vi "CoreState_Init.vi"(8 "error in (no error)":errorcluster, 11 "launcher in":refnum<class "launcher.lvclass">) -> (0 "error out":errorcluster, 3 "launcher out":refnum<class "launcher.lvclass">)   [LabVIEW 2021, in "launcher.lvclass"]
uses:
  launcher.lvclass
  TypeDefs/dvr_type.ctl
  _PARMS.ctl
  <userlib>/S2 Labs/Module Framework/Modules/Base/Launch Module Typdef.ctl
  <userlib>/S2 Labs/Module Framework/Modules/Base/Launch Module Parms.ctl
  launcher.lvclass/launcher.ctl
  <userlib>/S2 Labs/Module Framework/Modules/Base/Module.lvclass
  <userlib>/S2 Labs/Alarms and Events Toolkit/Alarms/Alarms Events.lvclass
  <vilib>/nisyscfg/nisyscfg.lvlib
  <resource>/objmgr/nisysapi.rc
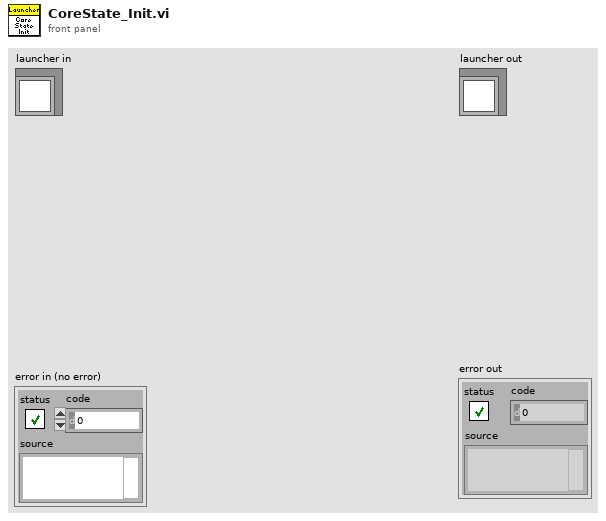
[diagram p1: front panel]
types:
  T1 = typedef "launcher.lvclass/dvr_type.ctl" = cluster{"_PARMS":T2}
  T2 = typedef "launcher.lvclass/_PARMS.ctl" = cluster{"ch_alias":string[], "ch_units":string[], "Modules to Launch":T3[]}
  T3 = typedef "Module.lvclass/Launch Module Typdef.ctl" = cluster{"Module":string, "Parameters":T4}
  T4 = typedef "Module.lvclass/Launch Module Parms.ctl" = cluster{"Name":string, "Arguments":string[], "Show FP?":bool}
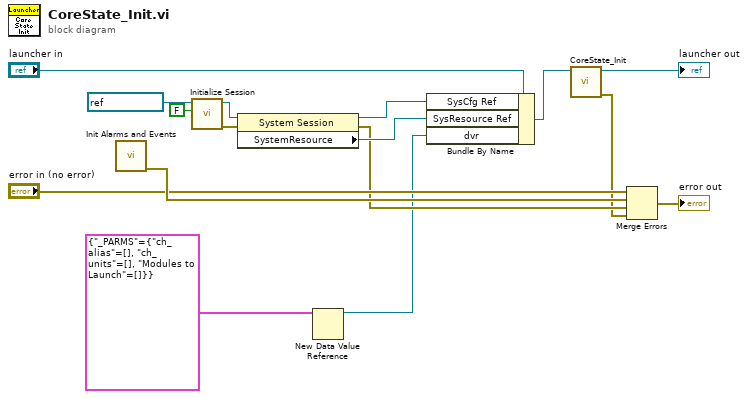
[diagram p0: block diagram]
diagram:
  n1 = call <userlib>:"Init Alarms and Events.vi"() -> ("error out"=w14:errorcluster)  [unwired: 11 in]
  n2 = call <vilib>:"Initialize Session.vi"("Force Property Refresh (T)"=FALSE, "Target (localhost)"=refnum<k21> "localhost") -> ("error out"=w12:errorcluster, "Session out"=w11:refnum<k21>)  [unwired: 8 in]
  n3 = property class="System Session"(reference=w11, error in=w12) -> (reference out=w6:refnum<k21>, error out=w4:errorcluster, "SystemResource"=w5:refnum<k20>)
  n4 = New Data Value Reference(data value=T1 {"_PARMS"={"ch_alias"=[], "ch_units"=[], "Modules to Launch"=[]}} ("dvr type")) -> (data value reference=w1:refnum<data-value>)  [unwired: 1 in, 1 out]
  n5 = Bundle By Name(cluster="launcher in", "SysCfg Ref"=w6, "SysResource Ref"=w5, "dvr"=w1) -> (w7:refnum<class "launcher.lvclass">)
  n6 = call-parent "CoreState_Init.vi"("Module in"=w7) -> ("error out"=w3:errorcluster, "Module out"=→"launcher out":refnum<class "launcher.lvclass">)  [unwired: 9 in]
  n7 = Merge Errors("error in (no error)", w14, w4, w3) -> (→"error out":errorcluster)
